vi "Graph.vi"(8 "error in (no error)":errorcluster, 10 "notifier out":refnum<notifier>, 11 "State in":T1={"State"=enum."Idle", "Start Time"=timestamp(0 s since 1904-01-01), "Configuration"={"Cycle Period"=0.0, "Setpoint Entry"=0.0, "Output Device"=enum."Huber Ministat 230", "Huber Ministat 230 Settings"={"VISA resource name"="", "Simulated?"=FALSE}, "Lauda Settings"={"VISA resource name"="", "Simulated?"=FALSE, "Pump Power"=2}, "Julabo FP-50 Settings"={"VISA resource name"="", "Simulated?"=FALSE, "Pump Power"=2}, "Internal Control?"=FALSE, "Huber Unistat 410 Settings"={"VISA resource name"="", "Simulated?"=FALSE}}, "Current Time"=timestamp(0 s since 1904-01-01), "First Iteration"=FALSE, "Data"={"TCU Speed"=0.0, "Temperature"=0.0}, "Process Name"="", "TCU On?"=FALSE, "Output Error"=FALSE, "Start Log"=FALSE, "Power Level Changed"=FALSE} {"Configuration"."Julabo FP-50 Settings"."Pump Power" min=0 max=8 step=1; "Configuration"."Lauda Settings"."Pump Power" min=0 max=8 step=1}) -> (0 "error out":errorcluster, 3 "State out":T1={"State"=enum."Idle", "Start Time"=timestamp(0 s since 1904-01-01), "Configuration"={"Cycle Period"=0.0, "Setpoint Entry"=0.0, "Output Device"=enum."Huber Ministat 230", "Huber Ministat 230 Settings"={"VISA resource name"="", "Simulated?"=FALSE}, "Lauda Settings"={"VISA resource name"="", "Simulated?"=FALSE, "Pump Power"=2}, "Julabo FP-50 Settings"={"VISA resource name"="", "Simulated?"=FALSE, "Pump Power"=2}, "Internal Control?"=FALSE, "Huber Unistat 410 Settings"={"VISA resource name"="", "Simulated?"=FALSE}}, "Current Time"=timestamp(0 s since 1904-01-01), "First Iteration"=FALSE, "Data"={"TCU Speed"=0.0, "Temperature"=0.0}, "Process Name"="", "TCU On?"=FALSE, "Output Error"=FALSE, "Start Log"=FALSE, "Power Level Changed"=FALSE} {"Configuration"."Julabo FP-50 Settings"."Pump Power" min=0 max=8 step=1; "Configuration"."Lauda Settings"."Pump Power" min=0 max=8 step=1})   [LabVIEW 2018, in "TCU Module.lvlib" / "TCU Module Engine.lvlib"]
uses:
  TCU Module Engine.lvlib
  TCU State Cluster.ctl
  State Enum.ctl
  TCU Module Settings Cluster.ctl
  Output Devices.ctl
  Huber TCU/Huber Settings.ctl
  Lauda Integral XT-150 TCU/Lauda Settings.ctl
  Julabo Type 1 TCU/Julabo Type 1 TCU Folder/Julabo FP-50 Settings.ctl
  Huber Unistat 410 TCU/Huber Unistat 410 Settings.ctl
  TCU Module.lvlib
  Huber TCU/Huber Ministat 230 TCU.lvlib
  Lauda Integral XT-150 TCU/Lauda TCU.lvlib
  Julabo Type 1 TCU/Julabo Type 1 TCU Folder/Julabo Type FP-50 TCU.lvlib
  Huber Unistat 410 TCU/Huber Unistat 410 TCU.lvlib
panel:
  # "Output Instruments"
  # "Output Instruments"
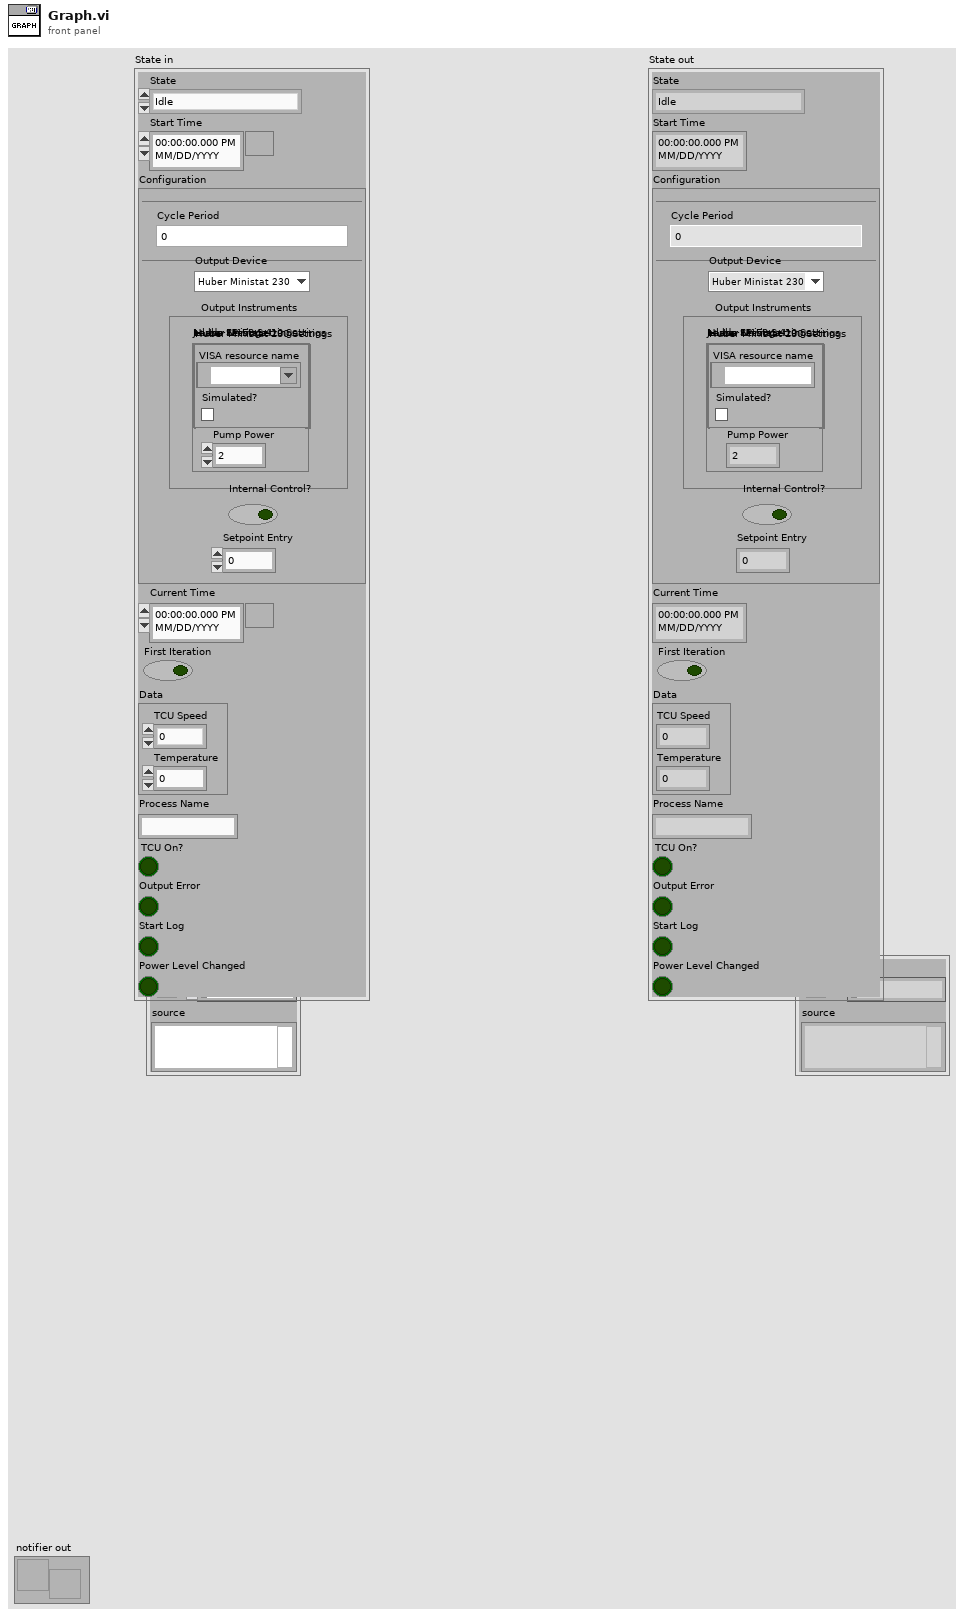
[diagram p1: front panel]
types:
  T1 = typedef "TCU Module.lvlib/TCU Module Engine.lvlib/TCU State Cluster.ctl" = cluster{"State":T2, "Start Time":timestamp, "Configuration":T3, "Current Time":timestamp, "First Iteration":bool, "Data":cluster{"TCU Speed":dbl, "Temperature":dbl}, "Process Name":string, "TCU On?":bool, "Output Error":bool, "Start Log":bool, "Power Level Changed":bool}
  T2 = typedef "TCU Module.lvlib/TCU Module Engine.lvlib/State Enum.ctl" = enum16{"Measuring", "Idle", "Paused"}
  T3 = typedef "TCU Module.lvlib/TCU Module Settings Cluster.ctl" = cluster{"Cycle Period":dbl, "Setpoint Entry":dbl, "Output Device":T4, "Huber Ministat 230 Settings":T5, "Lauda Settings":T6, "Julabo FP-50 Settings":T7, "Internal Control?":bool, "Huber Unistat 410 Settings":T8}
  T4 = typedef "Output Devices.ctl" = enum16{"Default", "Huber Ministat 230", "Huber Unistat 410", "Lauda XT-150", "Julabo FP-50"}
  T5 = typedef "Huber Ministat 230 TCU.lvlib/Huber Settings.ctl" = cluster{"VISA resource name":refnum<visa-resource-name>, "Simulated?":bool}
  T6 = typedef "Lauda TCU.lvlib/Lauda Settings.ctl" = cluster{"VISA resource name":refnum<visa-resource-name>, "Simulated?":bool, "Pump Power":i32}
  T7 = typedef "Julabo Type FP-50 TCU.lvlib/Julabo FP-50 Settings.ctl" = cluster{"VISA resource name":refnum<visa-resource-name>, "Simulated?":bool, "Pump Power":i32}
  T8 = typedef "Huber Unistat 410 TCU.lvlib/Huber Unistat 410 Settings.ctl" = cluster{"VISA resource name":refnum<visa-resource-name>, "Simulated?":bool}
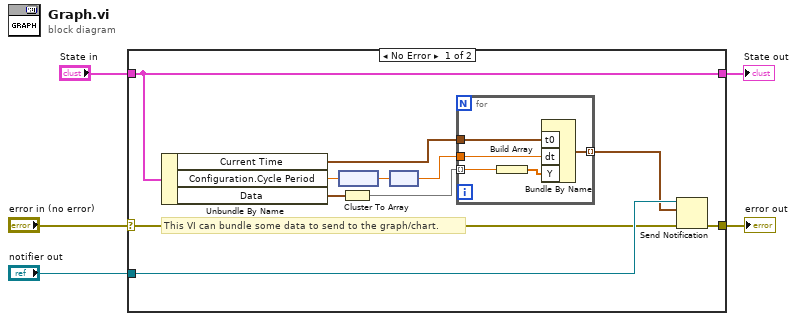
[diagram p0: block diagram]
diagram:
  n1 = case shown="No Error" "error in (no error)" {
    selector: "error in (no error)" -> [w13 w23]
    tunnel: [w12 w23] -> w4
    tunnel: "State in" -> [w16 w22]
    tunnel: [w16 w22] -> w2
    tunnel: "notifier out" -> [w14 _]
    frame No Error {
      # "This VI can bundle some data to send to the graph/chart."
      n2 = Unbundle By Name(w16) -> ("Current Time"=w11:timestamp, "Configuration.Cycle Period"=w10:dbl, "Data"=w15:cluster{"TCU Speed":dbl, "Temperature":dbl})
      n3 = node(w10) -> (w9:dbl[unit])
      n4 = Cluster To Array(cluster=w15) -> (array=w7:dbl[])
      n5 = node(w9) -> (w8:dbl)
      n6 = for {
        tunnel: w11 -> [w21]
        tunnel: w8 -> [w20]
        tunnel: w7 -> [w19] mode=indexing
        tunnel: [w17] -> w6 mode=indexing
        n7 = Build Array(w19) -> (w18:dbl[])
        n8 = Bundle By Name("t0"=w21, "dt"=w20, "Y"=w18) -> (w17:waveform(dbl))  [unwired: 1 in]
      }
      n9 = Send Notification(notification=w6, notifier=w14, error in (no error)=w13) -> (error out=w12:errorcluster)  [unwired: 1 out]
    }
    frame Error {
    }
  }
  "error out" <- w4
  "State out" <- w2
